vi "FPGA_Main.vi"   [LabVIEW 2016]
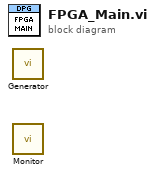
[diagram p0: block diagram]
diagram:
  n1 = call "Generator.vi"() -> ()  [unwired: 12 in]
  n2 = call "Monitor.vi"() -> ()  [unwired: 12 in]
